vi "test_Write Digital PWM Out.vi"(8 "error in (no error)":errorcluster, 11 "TestCase in":refnum<class "FPGA Addon Speciality IO Tests.lvclass">=refnum) -> (0 "error out":errorcluster, 3 "TestCase out":refnum<class "FPGA Addon Speciality IO Tests.lvclass">)   [LabVIEW 2026, in "FPGA Addon Speciality IO Tests.lvclass"]
uses:
  FPGA Addon Speciality IO Tests.lvclass
  FPGA Addon Test Class/FPGA Addon Test Class.lvclass
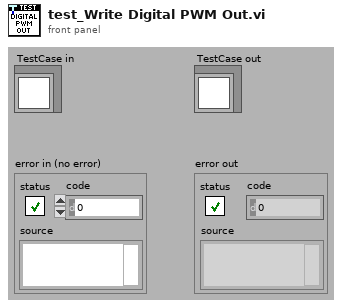
[diagram p1: front panel]
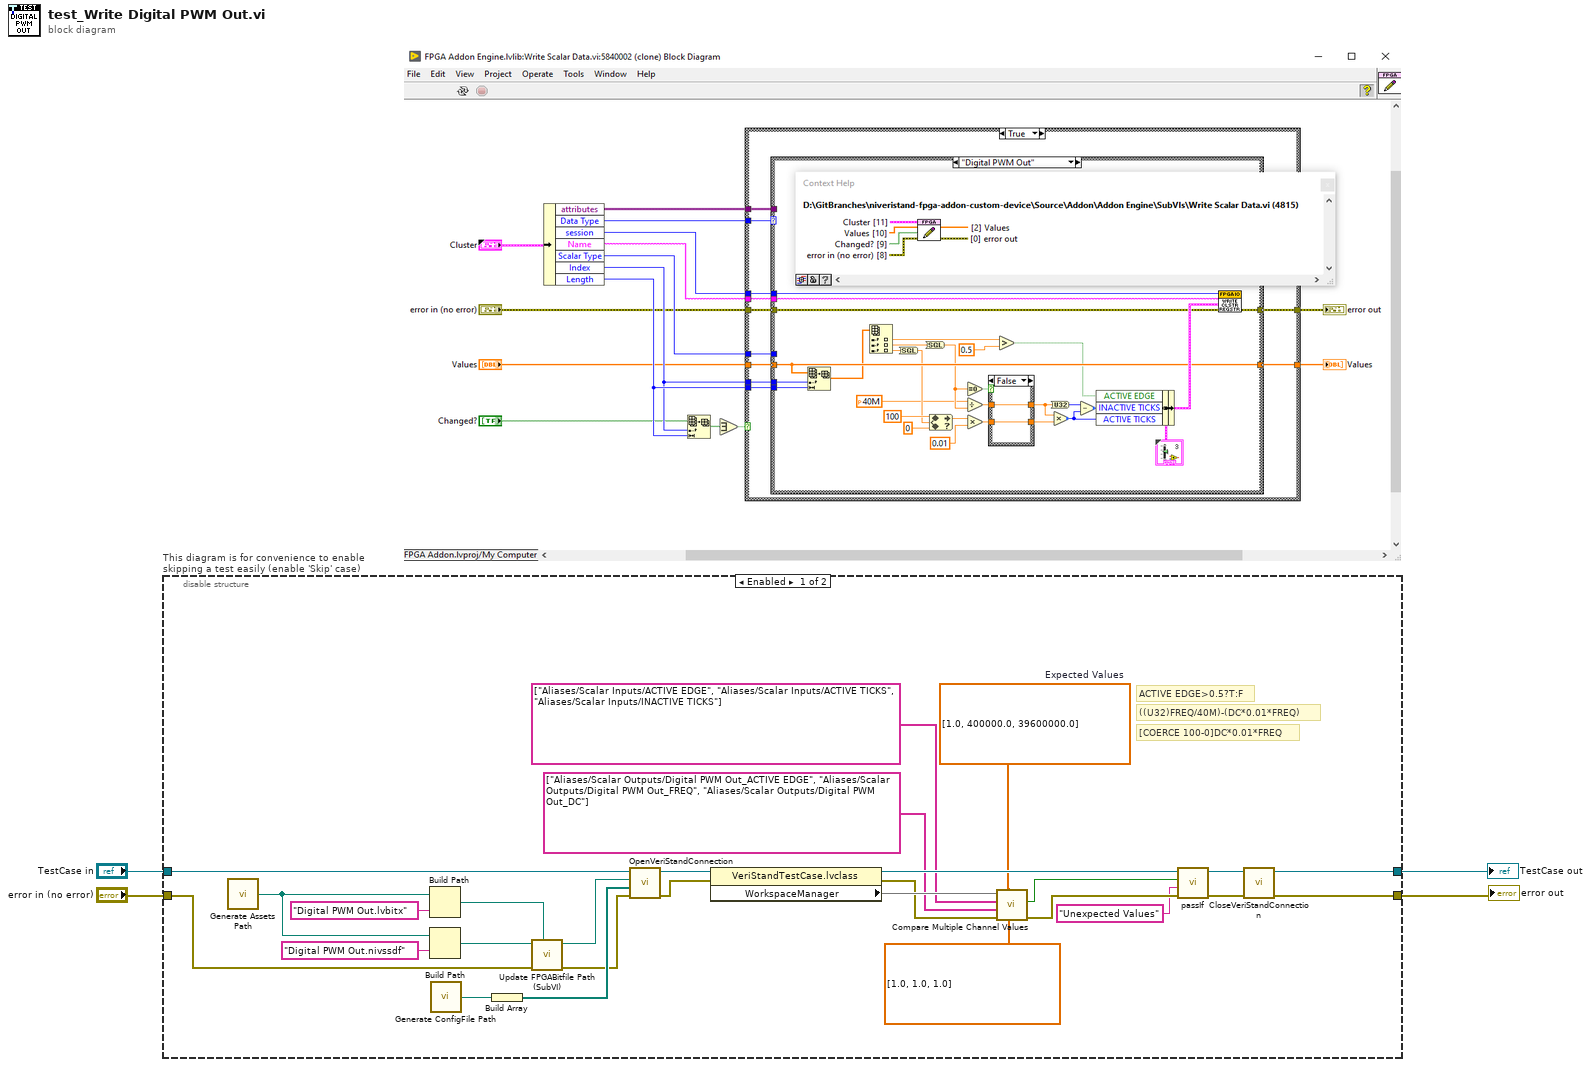
[diagram p0: block diagram]
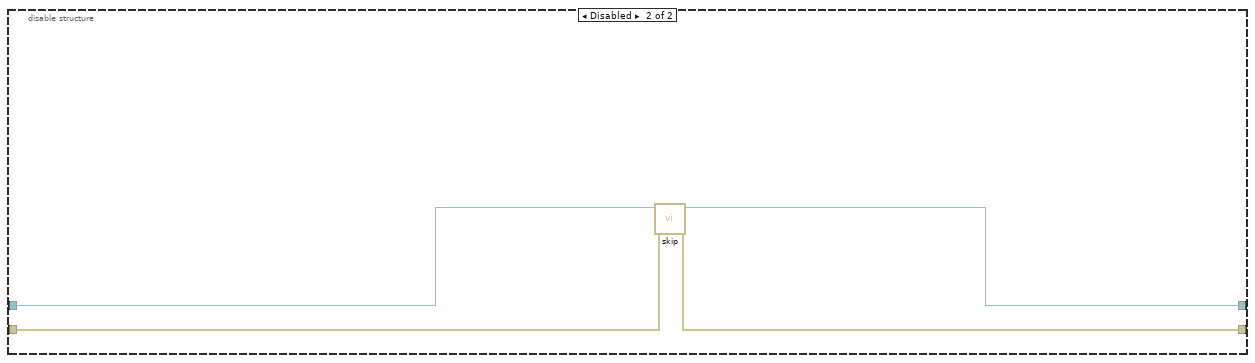
[diagram p2: hidden frame]
diagram:
  n1 = disable-structure "This diagram is for convenience to enable skipping a test easily (enable 'Skip' case)" shown="Enabled" {
    disable-tunnel: "TestCase in" -> [w29 w35]
    disable-tunnel: [w27 w33] -> w1
    disable-tunnel: [w28 w34] -> w3
    disable-tunnel: "error in (no error)" -> [w8 w32]
    frame Enabled {
      w18 = dbl[] [1.0, 400000.0, 39600000.0]  # Expected Values
      # "[COERCE 100-0]DC*0.01*FREQ"
      # "((U32)FREQ/40M)-(DC*0.01*FREQ)"
      # "ACTIVE EDGE>0.5?T:F"
      n2 = call "Generate Assets Path.vi"() -> ("Assets path"=w12:path)
      n3 = Build Path(base path=w12, name or relative path="Digital PWM Out.lvbitx") -> (appended path=w13:path)
      n4 = Build Path(base path=w12, name or relative path="Digital PWM Out.nivssdf") -> (appended path=w14:path)
      n5 = call "Generate ConfigFile Path.vi"() -> ("ConfigFile path"=w11:path)
      n6 = Build Array(w11) -> (w7:path[])
      n7 = call "Update FPGABitfile Path (SubVI).vi"("Bitfile Path"=w13, "error in (no error)"=w8, "System Definition path in"=w14) -> ("error out"=w6:errorcluster, "System Definition path out"=w5:path)  [unwired: 7 in]
      n8 = call-dynamic "OpenVeriStandConnection.vi"("error in (no error)"=w6, "overrides files"=w7, "System Definition File"=w5, "VeriStand Test Case in"=w29) -> ("error out"=w31:errorcluster, "VeriStand Test Case out"=w30:refnum<class "VeriStandTestCase.lvclass">)  [unwired: 5 in, 1 out]
      n9 = property class="VeriStandTestCase.lvclass"(reference=w30, error in=w31) -> (reference out=w26:refnum<class "VeriStandTestCase.lvclass">, error out=w22:errorcluster, "WorkspaceManager"=w23)
      n10 = call "Compare Multiple Channel Values.vi"("Values"=dbl[] [1.0, 1.0, 1.0], "Expected Values"=w18, "error in (no error)"=w22, "Scalar Outputs"=string[] ["Aliases/Scalar Outputs/Digital PWM Out_ACTIVE EDGE", "Aliases/Scalar Outputs/Digital PWM Out_FREQ", "Aliases/Scalar Outputs/Digital PWM Out_DC"] ("Channels"), "Scalar Inputs"=string[] ["Aliases/Scalar Inputs/ACTIVE EDGE", "Aliases/Scalar Inputs/ACTIVE TICKS", "Aliases/Scalar Inputs/INACTIVE TICKS"] ("Channels"), ".NET Refnum in"=w23) -> ("error out"=w17:errorcluster, "Equals?"=w16:bool)  [unwired: 4 in]
      n11 = call-dynamic "passIf.vi"("error in (no error)"=w17, "message (\"\")"="Unexpected Values" ("message (\"\")"), "pass"=w16, "TestCase in"=w26) -> ("error out"=w24:errorcluster, "TestCase out"=w25:refnum<class "FPGA Addon Speciality IO Tests.lvclass">)  [unwired: 6 in]
      n12 = call-dynamic "CloseVeriStandConnection.vi"("error in (no error)"=w24, "VeriStand Test Case in"=w25) -> ("error out"=w28:errorcluster, "VeriStand Test Case out"=w27:refnum<class "VeriStandTestCase.lvclass">)  [unwired: 8 in]
    }
    frame Disabled {
      # "skip test result while test is under development"
      n13 = call <vilib>:"skip.vi"("error in (no error)"=w32, "TestCase in"=w35) -> ("error out"=w34:errorcluster, "TestCase out"=w33:refnum<class "FPGA Addon Speciality IO Tests.lvclass">)  [unwired: 8 in]
    }
  }
  "error out" <- w3
  "TestCase out" <- w1
